vi "Pixels2Coordinates.vi"(5 "Y":dbl format="%#_13g", 7 "X":dbl format="%#_13g", 11 "Location (Pixel)":cluster{"X":sgl, "Y":sgl}={"X"=3.0, "Y"=4.0}) -> (3 "output cluster":cluster{"X":sgl, "Y":sgl})   [LabVIEW 2016]
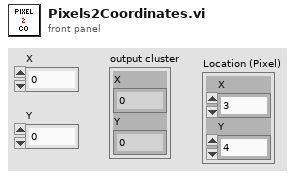
[diagram p1: front panel]
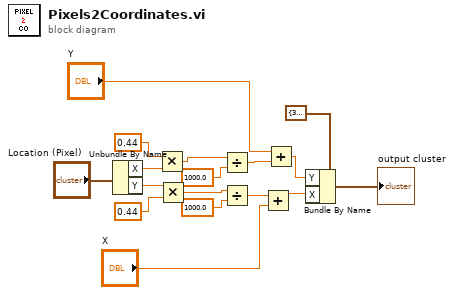
[diagram p0: block diagram]
diagram:
  n1 = Unbundle By Name("Location (Pixel)") -> ("X"=w14:sgl, "Y"=w12:sgl)
  n2 = Multiply(x=0.44, y=w14) -> (x*y=w11:dbl)
  n3 = Multiply(x=w12, y=0.44) -> (x*y=w9:dbl)
  n4 = Divide(x=w11, y=1000.0) -> (x/y=w6:dbl)
  n5 = Divide(x=w9, y=1000.0) -> (x/y=w3:dbl)
  n6 = Add(x=w3, y="X") -> (x+y=w2:dbl)
  n7 = Add(x="Y", y=w6) -> (x+y=w5:dbl)
  n8 = Bundle By Name(cluster=cluster{"X":sgl, "Y":sgl} {"X"=3.0, "Y"=4.0} ("Location (Pixel)"), "Y"=w5, "X"=w2) -> (→"output cluster":cluster{"X":sgl, "Y":sgl})
